vi "OAT Cascade Plot Indicator.vi"() -> ()   [LabVIEW 2017]
doc: "Uses the Cascade Plot to display the results of the spectral map as a function of rotational speed on a customized waveform graph."
uses:
  <vilib>/addons/Sound and Vibration/Order Analysis/Backward Compatibility/SubVIs/OAT Cascade Plot.ctl
panel:
  out "Cascade Plot":T1
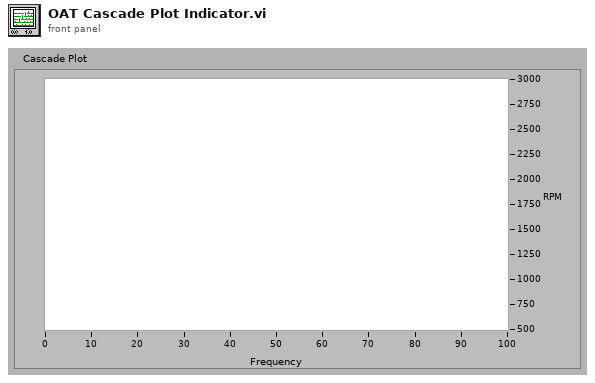
[diagram p1: front panel]
types:
  T1 = typedef "OAT Cascade Plot.ctl" = cluster{"X0":dbl, "dX":dbl, "Y":dbl[]}[]
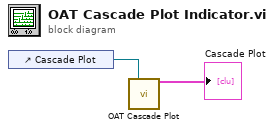
[diagram p0: block diagram]
diagram:
  n1 = control-ref of="Cascade Plot"() -> (w2:refnum<vi>)
  n2 = call <vilib>:"OAT Cascade Plot.vi"("cascade plot ref"=w2) -> ("cascade plot"=→"Cascade Plot":T1)  [unwired: 13 in, 1 out]
